vi "GetShutdown.vi"(8 "error in (no error)":errorcluster) -> (0 "error out":errorcluster, 2 "Shutdown":bool)   [LabVIEW 2023, in "Server.lvclass"]
doc: "Returns whether or not the Server should shut down. Also called internally in Listen.vi"
uses:
  Server.lvclass
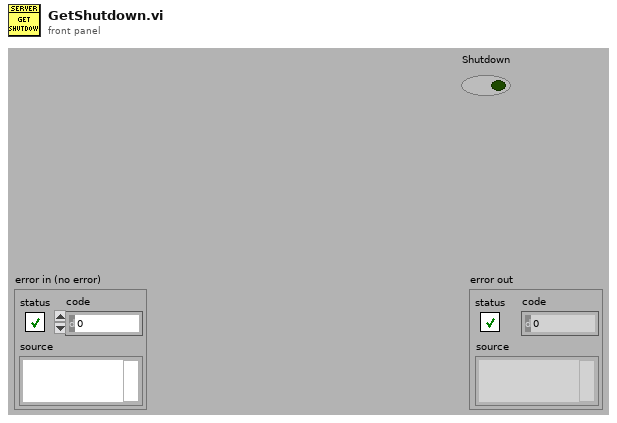
[diagram p1: front panel]
types:
  T1 = typedef "Server.lvclass/ObjectAttributes.ctl" = cluster{"Static Data":path, "MIME Types":variant, "Shutdown":bool, "API Queue":refnum<queue>, "ControlEndpoints":map{string, cluster{"Ref":refnum<vi>, "Mode":T2}}, "EventEndpoints":map{string, refnum<user-event>}}
  T2 = typedef "Server.lvclass/Control Ref Endpoint Access Mode.ctl" = enum16{"None", "Read/Write", "Read Only", "Write Only"}
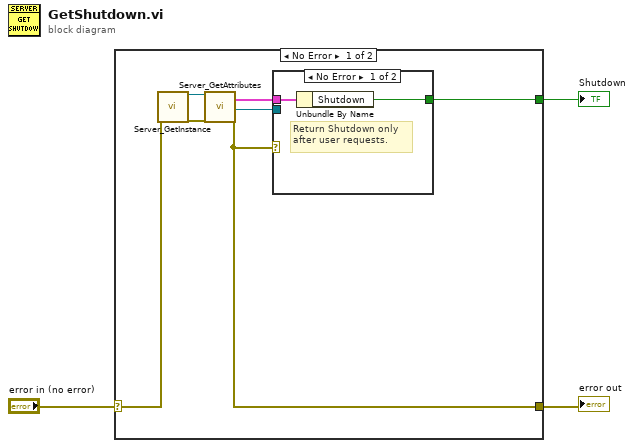
[diagram p0: block diagram]
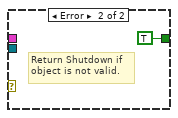
[diagram p2: hidden frame]
diagram:
  n1 = case shown="No Error" "error in (no error)" {
    selector: "error in (no error)" -> [w7 w14]
    tunnel: [w5 w14] -> w2
    tunnel: [w9 _] -> w1
    frame No Error {
      n2 = call "Server_GetInstance.vi"("error in (no error)"=w7) -> ("reference out"=w8:refnum<class "Server.lvclass">, "error out"=w6:errorcluster)  [unwired: 14 in, 3 out]
      n3 = call "Server_GetAttributes.vi"("reference in"=w8, "error in (no error)"=w6) -> ("Data"=w10:T1, "DataRef"=w4:refnum<data-value>, "error out"=w5:errorcluster)  [unwired: 14 in, 1 out]
      n4 = case shown="No Error" w5 {
        tunnel: w10 -> [w12 _]
        tunnel: [w11 TRUE ("Shutdown")] -> w9
        tunnel: w4 -> [_ _]
        frame No Error {
          # "Return Shutdown only\nafter user requests."
          n5 = Unbundle By Name(w12) -> ("Shutdown"=w11:bool)
        }
        frame Error {
          # "Return Shutdown if\nobject is not valid."
        }
      }
    }
    frame Error {
    }
  }
  "error out" <- w2
  "Shutdown" <- w1
